vi "XLP80_Globals_SettingsFix.vi"() -> ()   [LabVIEW 2021]
panel:
  out "INI File PathOption":enum16{"WindowsPath", "LocalPath", "Path"}(ring)=enum."LocalPath"
  out "InternalTimebaseHz":dbl=80000000.0 caption="Do not change!" format="%.2e"
  out "Settings VI":string="Globals_Settings_XLP80.vi"
  out "INI-File Name":string="XLP80.INI"
  # "Laser: 9.16V   = 40mm\n             1.16 V = -40mm\n             5.16 V = 0mm"
  # "Knüppel X: 1.596 mV/V * 5V =7.980V = 200N"
  # "Knüppel X: 1.556 mV/V * 5V =7.780V = 200N"
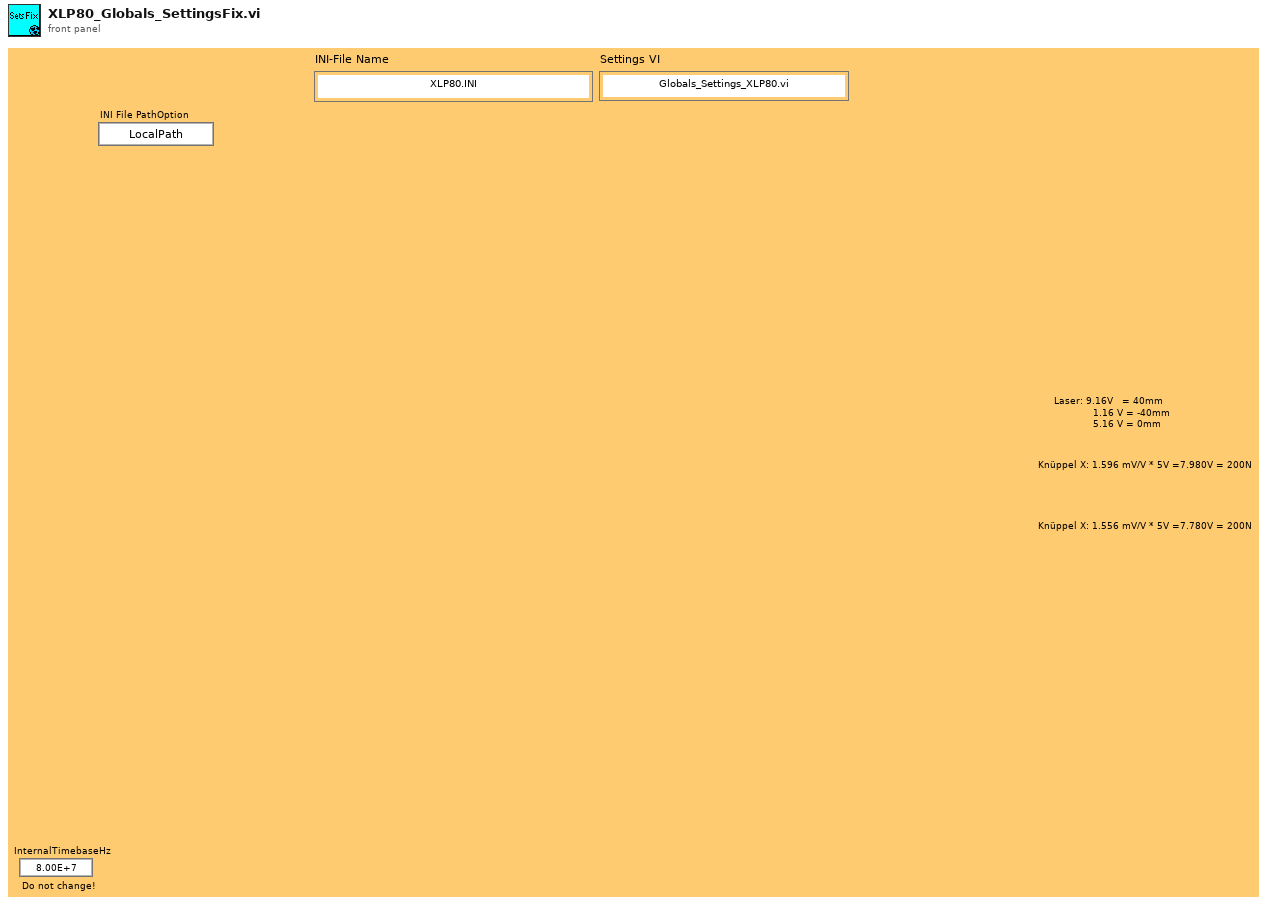
[diagram p1: front panel]
diagram:
